vi "_Open_data.vi"(0 "Documented VI path":path, 11 "error in":errorcluster) -> (8 "XML Info cluster":T1={"_vi_name_"="", "_vi_description_text_"="", "_vi_controls_and_indicators_descriptions_"="", "_name_of_owning_library_"="", "_owning_library_html_"="", "_Packages_"="Base Package", "_Platforms_"="Windows", "_details_text_"="Put details here", "_example_screenshot_"="", "_example_vi_"="", "_path_to_example_file_"=path "", "IsDetailsON?"=FALSE, "IsOwningLibraryON?"=FALSE, "IsExamplesON?"=FALSE, "IsTableON?"=FALSE, "IsScrollableON?"=FALSE, "IsDetailedHelpLinkON?"=FALSE, "Table Objects array"=[], "Table Descriptions array"=[], "Table Links array"=[], "Start path location"=enum."VI folder"}, 15 "error out":errorcluster)   [LabVIEW 2012]
uses:
  _Controls and TypeDefs/InfoFromOldHTML_cluster.ctl
  _Controls and TypeDefs/StartPathLocation_enum.ctl
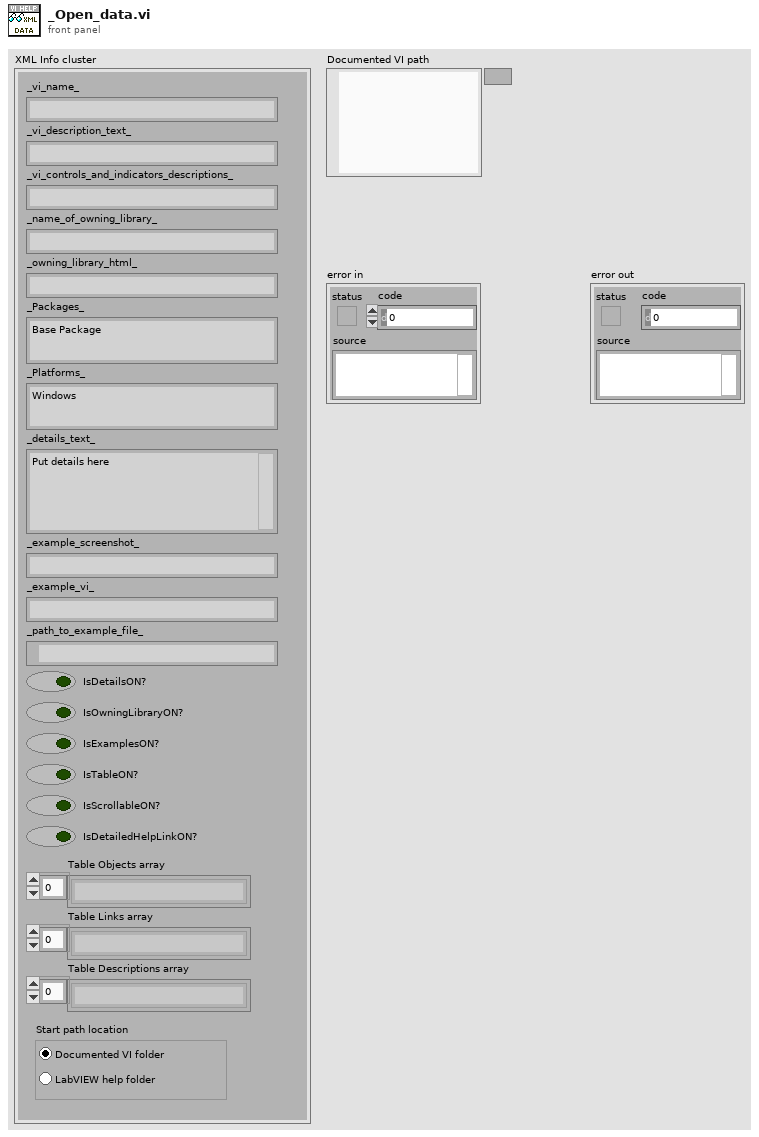
[diagram p1: front panel]
types:
  T1 = typedef "InfoFromOldHTML_cluster.ctl" = cluster{"_vi_name_":string, "_vi_description_text_":string, "_vi_controls_and_indicators_descriptions_":string, "_name_of_owning_library_":string, "_owning_library_html_":string, "_Packages_":string, "_Platforms_":string, "_details_text_":string, "_example_screenshot_":string, "_example_vi_":string, "_path_to_example_file_":path, "IsDetailsON?":bool, "IsOwningLibraryON?":bool, "IsExamplesON?":bool, "IsTableON?":bool, "IsScrollableON?":bool, "IsDetailedHelpLinkON?":bool, "Table Objects array":string[], "Table Descriptions array":string[], "Table Links array":string[], "Start path location":T2}
  T2 = typedef "StartPathLocation_enum.ctl" = enum32{"VI folder", "Help folder"}
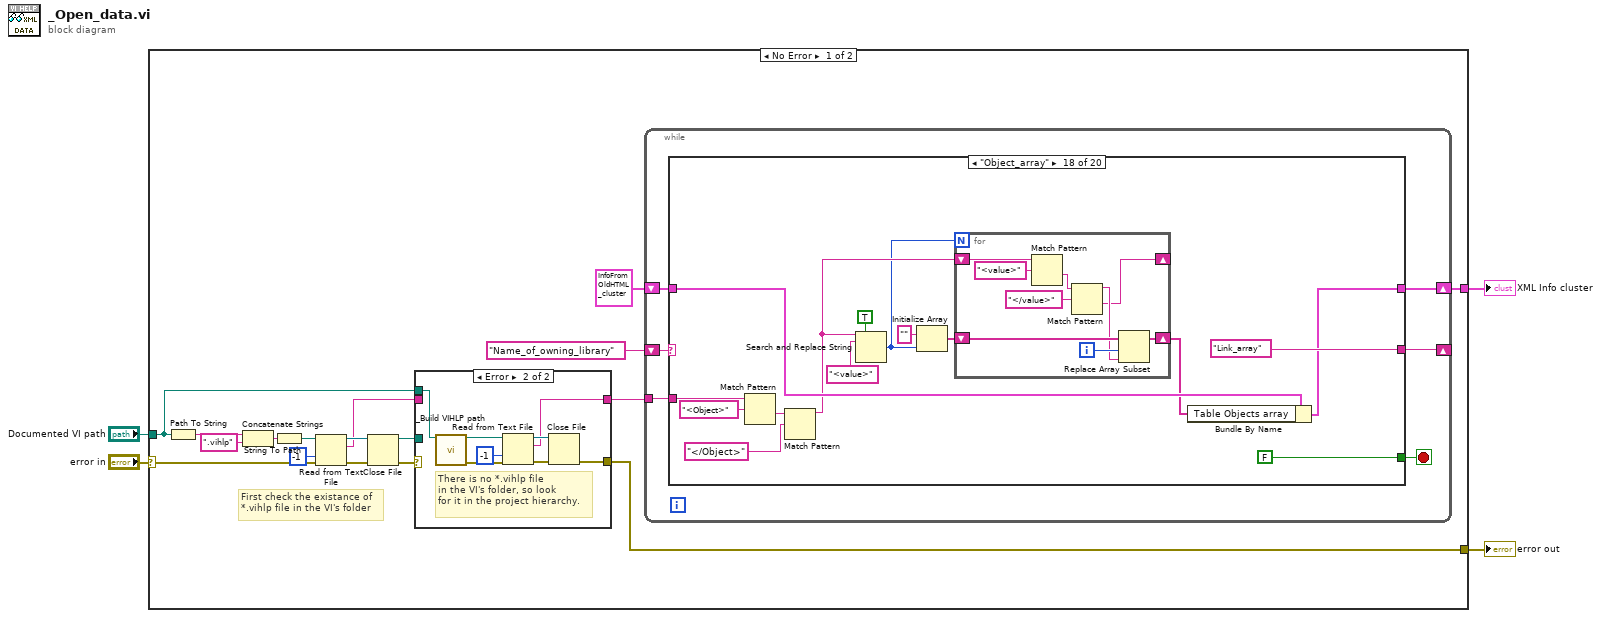
[diagram p0: block diagram]
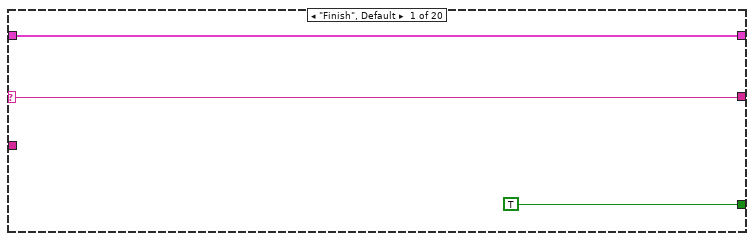
[diagram p3: hidden frame]
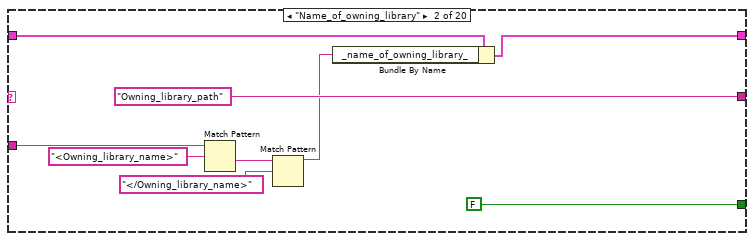
[diagram p4: hidden frame]
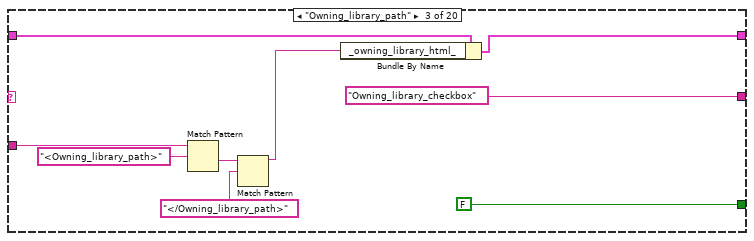
[diagram p5: hidden frame]
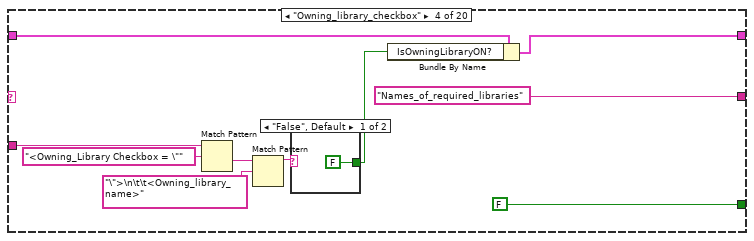
[diagram p6: hidden frame]
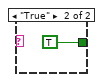
[diagram p7: hidden frame]
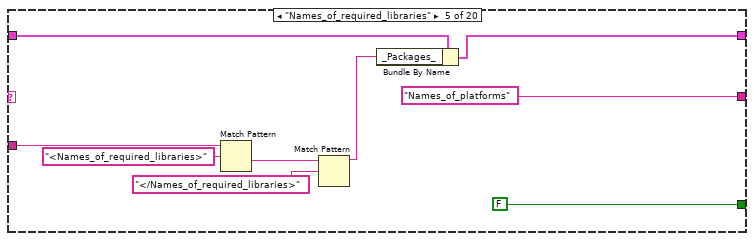
[diagram p8: hidden frame]
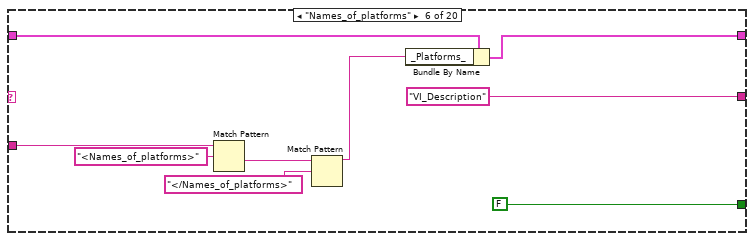
[diagram p9: hidden frame]
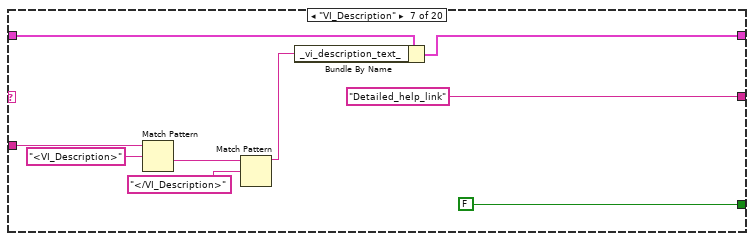
[diagram p10: hidden frame]
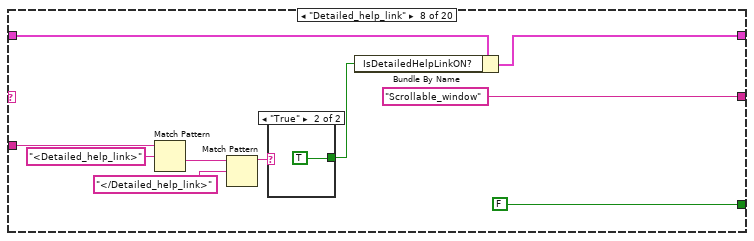
[diagram p11: hidden frame]
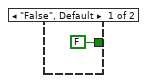
[diagram p12: hidden frame]
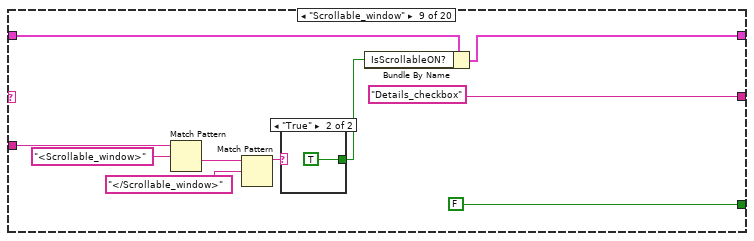
[diagram p13: hidden frame]
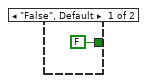
[diagram p14: hidden frame]
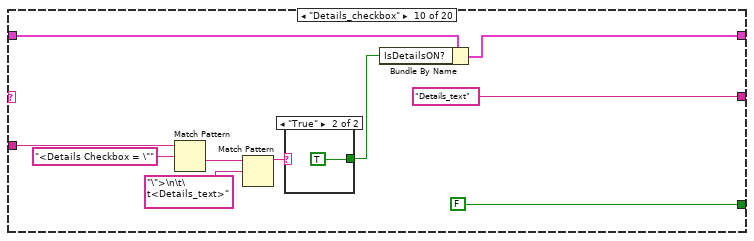
[diagram p15: hidden frame]
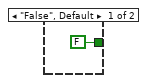
[diagram p16: hidden frame]
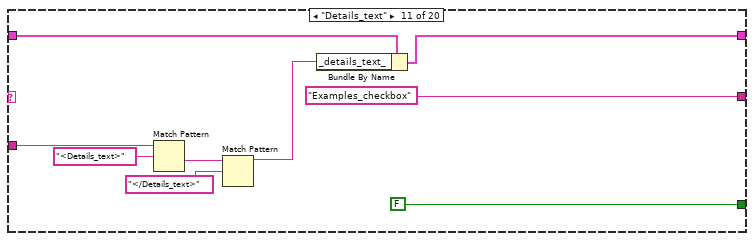
[diagram p17: hidden frame]
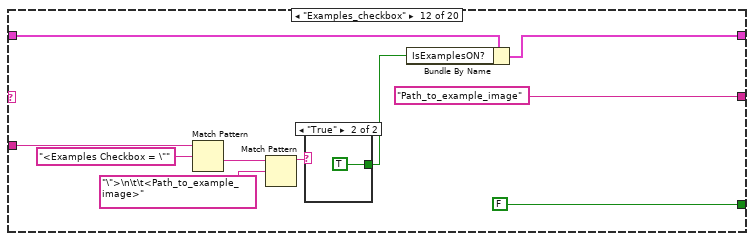
[diagram p18: hidden frame]
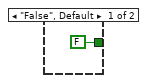
[diagram p19: hidden frame]
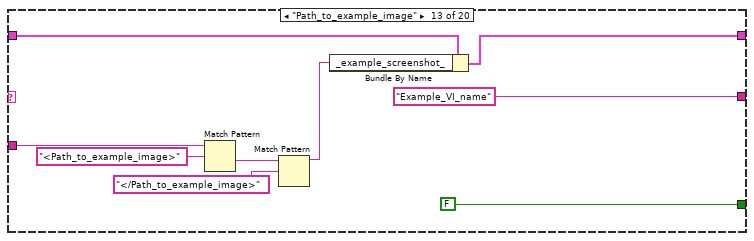
[diagram p20: hidden frame]
diagram:
  n1 = case shown="No Error" "error in" {
    selector: "error in" -> [w5 w280]
    tunnel: [w16 T1 {"_vi_name_"="", "_vi_description_text_"="", "_vi_controls_and_indicators_descriptions_"="", "_name_of_owning_library_"="", "_owning_library_html_"="", "_Packages_"="Base Package", "_Platforms_"="Windows", "_details_text_"="Put details here", "_example_screenshot_"="", "_example_vi_"="", "_path_to_example_file_"=path "", "IsDetailsON?"=FALSE, "IsOwningLibraryON?"=FALSE, "IsExamplesON?"=FALSE, "IsTableON?"=FALSE, "IsScrollableON?"=FALSE, "IsDetailedHelpLinkON?"=FALSE, "Table Objects array"=[], "Table Descriptions array"=[], "Table Links array"=[], "Start path location"=enum."VI folder"} ("Info extracted from old HTML")] -> w4
    tunnel: [w8 w280] -> w3
    tunnel: "Documented VI path" -> [w6 _]
    frame No Error {
      # "First check the existance of\n*.vihlp file in the VI's folder"
      n2 = Path To String(path=w6) -> (string=w15:string)
      n3 = Concatenate Strings(w15, ".vihlp" ("string")) -> (w13:string)
      n4 = String To Path(string=w13) -> (path=w7:path)
      n5 = Read from Text File(file (use dialog)=w7, count=-1, error in=w5) -> (refnum out=w20:refnum<file>, text=w10:string, error out=w21:errorcluster)  [unwired: 1 in, 1 out]
      n6 = Close File(refnum=w20, error in=w21) -> (path=w11:path, error out=w12:errorcluster)
      n7 = case shown="Error" w12 {
        selector: w12 -> [w22 _]
        tunnel: w11 -> [_ _]
        tunnel: w10 -> [w23 _]
        tunnel: [w23 w25] -> w9
        tunnel: [w22 w26] -> w8
        tunnel: w6 -> [_ w24]
        frame No Error {
          # "No error, such *.vihlp file\nexists in the VI's folder"
        }
        frame Error {
          # "There is no *.vihlp file\nin the VI's folder, so look\nfor it in the project hierarchy."
          n8 = call "_Build VIHLP path.vi"("Documented VI path"=w24) -> ("Path to VIHLP file"=w28:path, "error out"=w29:errorcluster)  [unwired: 13 in]
          n9 = Read from Text File(file (use dialog)=w28, count=-1, error in=w29) -> (refnum out=w27:refnum<file>, text=w25:string, error out=w31:errorcluster)  [unwired: 1 in, 1 out]
          n10 = Close File(refnum=w27, error in=w31) -> (error out=w26:errorcluster)  [unwired: 1 out]
        }
      }
      n11 = while {
        shift-right: [w34] -> _
        shift-left: "Name_of_owning_library" -> [w36]
        tunnel: w9 -> [w37]
        shift-right: [w32] -> w16
        shift-left: T1 {"_vi_name_"="", "_vi_description_text_"="", "_vi_controls_and_indicators_descriptions_"="", "_name_of_owning_library_"="", "_owning_library_html_"="", "_Packages_"="Base Package", "_Platforms_"="Windows", "_details_text_"="Put details here", "_example_screenshot_"="", "_example_vi_"="", "_path_to_example_file_"=path "", "IsDetailsON?"=FALSE, "IsOwningLibraryON?"=FALSE, "IsExamplesON?"=FALSE, "IsTableON?"=FALSE, "IsScrollableON?"=FALSE, "IsDetailedHelpLinkON?"=FALSE, "Table Objects array"=[], "Table Descriptions array"=[], "Table Links array"=[], "Start path location"=enum."VI folder"} ("Info extracted from old HTML") -> [w35]
        stop <- w33 stop-if-true
        n12 = case shown="\"Object_array\"" w36 {
          selector: w36 -> [w39 _ _ _ _ _ _ _ _ _ _ _ _ _ _ _ _ _ _ _]
          tunnel: w37 -> [_ w45 w54 w64 w75 w84 w94 w104 w116 w128 w139 w149 w160 w169 w179 w189 w201 w218 w232 w257]
          tunnel: w35 -> [w38 w43 w52 w62 w73 w82 w91 w101 w113 w125 w136 w146 w157 w166 w176 w186 w198 w215 w233 w256]
          tunnel: [w39 "Owning_library_path" "Owning_library_checkbox" "Names_of_required_libraries" "Names_of_platforms" "VI_Description" "Detailed_help_link" "Scrollable_window" "Details_checkbox" "Details_text" "Examples_checkbox" "Path_to_example_image" "Example_VI_name" "Example_VI_path" "Start_path" "Table_checkbox" "Object_array" "Link_array" "Description_array" "Finish"] -> w34
          tunnel: [TRUE FALSE FALSE FALSE FALSE FALSE FALSE FALSE FALSE FALSE FALSE FALSE FALSE FALSE FALSE FALSE FALSE FALSE FALSE FALSE] -> w33
          tunnel: [w38 w42 w51 w61 w72 w81 w90 w100 w112 w124 w135 w145 w156 w165 w175 w185 w197 w214 w231 w255] -> w32
          frame "Finish", Default {
          }
          frame "Name_of_owning_library" {
            n13 = Match Pattern(string=w45, regular expression="<Owning_library_name>") -> (after substring=w47:string)  [unwired: 1 in, 3 out]
            n14 = Match Pattern(string=w47, regular expression="</Owning_library_name>") -> (before substring=w41:string)  [unwired: 1 in, 3 out]
            n15 = Bundle By Name(cluster=w43, "_name_of_owning_library_"=w41) -> (w42:T1)
          }
          frame "Owning_library_path" {
            n16 = Match Pattern(string=w54, regular expression="<Owning_library_path>") -> (after substring=w56:string)  [unwired: 1 in, 3 out]
            n17 = Match Pattern(string=w56, regular expression="</Owning_library_path>") -> (before substring=w50:string)  [unwired: 1 in, 3 out]
            n18 = Bundle By Name(cluster=w52, "_owning_library_html_"=w50) -> (w51:T1)
          }
          frame "Owning_library_checkbox" {
            n19 = Match Pattern(string=w64, regular expression="<Owning_Library Checkbox = \"") -> (after substring=w66:string)  [unwired: 1 in, 3 out]
            n20 = Match Pattern(string=w66, regular expression="\">\n\t\t<Owning_library_name>") -> (before substring=w60:string)  [unwired: 1 in, 3 out]
            n21 = case shown="\"False\", Default" w60 {
              tunnel: [FALSE TRUE] -> w59
              frame "False", Default {
              }
              frame "True" {
              }
            }
            n22 = Bundle By Name(cluster=w62, "IsOwningLibraryON?"=w59) -> (w61:T1)
          }
          frame "Names_of_required_libraries" {
            n23 = Match Pattern(string=w75, regular expression="<Names_of_required_libraries>") -> (after substring=w77:string)  [unwired: 1 in, 3 out]
            n24 = Match Pattern(string=w77, regular expression="</Names_of_required_libraries>") -> (before substring=w71:string)  [unwired: 1 in, 3 out]
            n25 = Bundle By Name(cluster=w73, "_Packages_"=w71) -> (w72:T1)
          }
          frame "Names_of_platforms" {
            n26 = Match Pattern(string=w84, regular expression="<Names_of_platforms>") -> (after substring=w86:string)  [unwired: 1 in, 3 out]
            n27 = Match Pattern(string=w86, regular expression="</Names_of_platforms>") -> (before substring=w80:string)  [unwired: 1 in, 3 out]
            n28 = Bundle By Name(cluster=w82, "_Platforms_"=w80) -> (w81:T1)
          }
          frame "VI_Description" {
            n29 = Match Pattern(string=w94, regular expression="<VI_Description>") -> (after substring=w96:string)  [unwired: 1 in, 3 out]
            n30 = Match Pattern(string=w96, regular expression="</VI_Description>") -> (before substring=w89:string)  [unwired: 1 in, 3 out]
            n31 = Bundle By Name(cluster=w91, "_vi_description_text_"=w89) -> (w90:T1)
          }
          frame "Detailed_help_link" {
            n32 = Match Pattern(string=w104, regular expression="<Detailed_help_link>") -> (after substring=w106:string)  [unwired: 1 in, 3 out]
            n33 = Match Pattern(string=w106, regular expression="</Detailed_help_link>") -> (before substring=w99:string)  [unwired: 1 in, 3 out]
            n34 = case shown="\"True\"" w99 {
              tunnel: [FALSE TRUE] -> w98
              frame "False", Default {
              }
              frame "True" {
              }
            }
            n35 = Bundle By Name(cluster=w101, "IsDetailedHelpLinkON?"=w98) -> (w100:T1)
          }
          frame "Scrollable_window" {
            n36 = Match Pattern(string=w116, regular expression="<Scrollable_window>") -> (after substring=w118:string)  [unwired: 1 in, 3 out]
            n37 = Match Pattern(string=w118, regular expression="</Scrollable_window>") -> (before substring=w111:string)  [unwired: 1 in, 3 out]
            n38 = case shown="\"True\"" w111 {
              tunnel: [FALSE TRUE] -> w110
              frame "False", Default {
              }
              frame "True" {
              }
            }
            n39 = Bundle By Name(cluster=w113, "IsScrollableON?"=w110) -> (w112:T1)
          }
          frame "Details_checkbox" {
            n40 = Match Pattern(string=w128, regular expression="<Details Checkbox = \"") -> (after substring=w130:string)  [unwired: 1 in, 3 out]
            n41 = Match Pattern(string=w130, regular expression="\">\n\t\t<Details_text>") -> (before substring=w123:string)  [unwired: 1 in, 3 out]
            n42 = case shown="\"True\"" w123 {
              tunnel: [FALSE TRUE] -> w122
              frame "False", Default {
              }
              frame "True" {
              }
            }
            n43 = Bundle By Name(cluster=w125, "IsDetailsON?"=w122) -> (w124:T1)
          }
          frame "Details_text" {
            n44 = Match Pattern(string=w139, regular expression="<Details_text>") -> (after substring=w141:string)  [unwired: 1 in, 3 out]
            n45 = Match Pattern(string=w141, regular expression="</Details_text>") -> (before substring=w134:string)  [unwired: 1 in, 3 out]
            n46 = Bundle By Name(cluster=w136, "_details_text_"=w134) -> (w135:T1)
          }
          frame "Examples_checkbox" {
            n47 = Match Pattern(string=w149, regular expression="<Examples Checkbox = \"") -> (after substring=w151:string)  [unwired: 1 in, 3 out]
            n48 = Match Pattern(string=w151, regular expression="\">\n\t\t<Path_to_example_image>") -> (before substring=w144:string)  [unwired: 1 in, 3 out]
            n49 = case shown="\"True\"" w144 {
              tunnel: [FALSE TRUE] -> w143
              frame "False", Default {
              }
              frame "True" {
              }
            }
            n50 = Bundle By Name(cluster=w146, "IsExamplesON?"=w143) -> (w145:T1)
          }
          frame "Path_to_example_image" {
            n51 = Match Pattern(string=w160, regular expression="<Path_to_example_image>") -> (after substring=w162:string)  [unwired: 1 in, 3 out]
            n52 = Match Pattern(string=w162, regular expression="</Path_to_example_image>") -> (before substring=w155:string)  [unwired: 1 in, 3 out]
            n53 = Bundle By Name(cluster=w157, "_example_screenshot_"=w155) -> (w156:T1)
          }
          frame "Example_VI_name" {
            n54 = Match Pattern(string=w169, regular expression="<Example_VI_name>") -> (after substring=w171:string)  [unwired: 1 in, 3 out]
            n55 = Match Pattern(string=w171, regular expression="</Example_VI_name>") -> (before substring=w164:string)  [unwired: 1 in, 3 out]
            n56 = Bundle By Name(cluster=w166, "_example_vi_"=w164) -> (w165:T1)
          }
          frame "Example_VI_path" {
            n57 = Match Pattern(string=w179, regular expression="<Example_VI_path>") -> (after substring=w181:string)  [unwired: 1 in, 3 out]
            n58 = Match Pattern(string=w181, regular expression="</Example_VI_path>") -> (before substring=w174:string)  [unwired: 1 in, 3 out]
            n59 = String To Path(string=w174) -> (path=w173:path)
            n60 = Bundle By Name(cluster=w176, "_path_to_example_file_"=w173) -> (w175:T1)
          }
          frame "Start_path" {
            n61 = Match Pattern(string=w189, regular expression="<Start_path>") -> (after substring=w191:string)  [unwired: 1 in, 3 out]
            n62 = Match Pattern(string=w191, regular expression="</Start_path>") -> (before substring=w184:string)  [unwired: 1 in, 3 out]
            n63 = case shown="\"LabVIEW_Help_folder\"" w184 {
              tunnel: [StartPathLocation_enum."VI folder" ("Start path location") StartPathLocation_enum."Help folder" ("Start path location")] -> w183
              frame "VI_folder", Default {
              }
              frame "LabVIEW_Help_folder" {
              }
            }
            n64 = Bundle By Name(cluster=w186, "Start path location"=w183) -> (w185:T1)
          }
          frame "Table_checkbox" {
            n65 = Match Pattern(string=w201, regular expression="<Table Checkbox = \"") -> (after substring=w203:string)  [unwired: 1 in, 3 out]
            n66 = Match Pattern(string=w203, regular expression="\">\n\t\t<Object>") -> (before substring=w196:string)  [unwired: 1 in, 3 out]
            n67 = case shown="\"True\"" w196 {
              tunnel: [FALSE TRUE] -> w195
              frame "False", Default {
              }
              frame "True" {
              }
            }
            n68 = Bundle By Name(cluster=w198, "IsTableON?"=w195) -> (w197:T1)
          }
          frame "Object_array" {
            n69 = Match Pattern(string=w218, regular expression="<Object>") -> (after substring=w220:string)  [unwired: 1 in, 3 out]
            n70 = Match Pattern(string=w220, regular expression="</Object>") -> (before substring=w213:string)  [unwired: 1 in, 3 out]
            n71 = Search and Replace String(replace all?=TRUE ("replace all? (F)"), input string=w213, search string="<value>") -> (number of replacements=w210:i32)  [unwired: 5 in, 3 out]
            n72 = Initialize Array("", w210) -> (w208:string[])
            n73 = for {
              N: w210 -> [_]
              shift-right: [w222] -> _
              shift-left: w213 -> [w230]
              shift-right: [w224] -> w207
              shift-left: w208 -> [w226]
              i -> [w225]
              n74 = Match Pattern(string=w230, regular expression="<value>") -> (after substring=w228:string)  [unwired: 1 in, 3 out]
              n75 = Match Pattern(string=w228, regular expression="</value>") -> (before substring=w223:string, after substring=w222:string)  [unwired: 1 in, 2 out]
              n76 = Replace Array Subset(array=w226, new element=w223, index=w225) -> (w224:string[])
            }
            n77 = Bundle By Name(cluster=w215, "Table Objects array"=w207) -> (w214:T1)
          }
          frame "Link_array" {
            n78 = Match Pattern(string=w232, regular expression="<Link>") -> (after substring=w235:string)  [unwired: 1 in, 3 out]
            n79 = Match Pattern(string=w235, regular expression="</Link>") -> (before substring=w237:string)  [unwired: 1 in, 3 out]
            n80 = Search and Replace String(replace all?=TRUE ("replace all? (F)"), input string=w237, search string="<value>") -> (number of replacements=w240:i32)  [unwired: 5 in, 3 out]
            n81 = Initialize Array("", w240) -> (w242:string[])
            n82 = for {
              N: w240 -> [_]
              shift-right: [w246] -> _
              shift-left: w237 -> [w254]
              shift-right: [w248] -> w243
              shift-left: w242 -> [w250]
              i -> [w249]
              n83 = Match Pattern(string=w254, regular expression="<value>") -> (after substring=w252:string)  [unwired: 1 in, 3 out]
              n84 = Match Pattern(string=w252, regular expression="</value>") -> (before substring=w247:string, after substring=w246:string)  [unwired: 1 in, 2 out]
              n85 = Replace Array Subset(array=w250, new element=w247, index=w249) -> (w248:string[])
            }
            n86 = Bundle By Name(cluster=w233, "Table Links array"=w243) -> (w231:T1)
          }
          frame "Description_array" {
            n87 = Match Pattern(string=w257, regular expression="<Description>") -> (after substring=w259:string)  [unwired: 1 in, 3 out]
            n88 = Match Pattern(string=w259, regular expression="</Description>") -> (before substring=w261:string)  [unwired: 1 in, 3 out]
            n89 = Search and Replace String(replace all?=TRUE ("replace all? (F)"), input string=w261, search string="<value>") -> (number of replacements=w264:i32)  [unwired: 5 in, 3 out]
            n90 = Initialize Array("", w264) -> (w266:string[])
            n91 = for {
              N: w264 -> [_]
              shift-right: [w270] -> _
              shift-left: w261 -> [w278]
              shift-right: [w272] -> w267
              shift-left: w266 -> [w274]
              i -> [w273]
              n92 = Match Pattern(string=w278, regular expression="<value>") -> (after substring=w276:string)  [unwired: 1 in, 3 out]
              n93 = Match Pattern(string=w276, regular expression="</value>") -> (before substring=w271:string, after substring=w270:string)  [unwired: 1 in, 2 out]
              n94 = Replace Array Subset(array=w274, new element=w271, index=w273) -> (w272:string[])
            }
            n95 = Bundle By Name(cluster=w256, "Table Descriptions array"=w267) -> (w255:T1)
          }
        }
      }
    }
    frame Error {
    }
  }
  "error out" <- w3
  "XML Info cluster" <- w4
